vi "pathsConfig.vi"(0 "TDMS file out path IN":path=path "", 5 "Background out path IN":path=path "", 11 "Error IN":errorcluster caption="constante d'erreur") -> (15 "Error OUT":errorcluster caption="constante d'erreur")   [LabVIEW 2020]
panel:
  in  "OK":bool
  out "Background out path":path
  out "TDMS file out path":path
  # "PATHS CONFIGURATION"
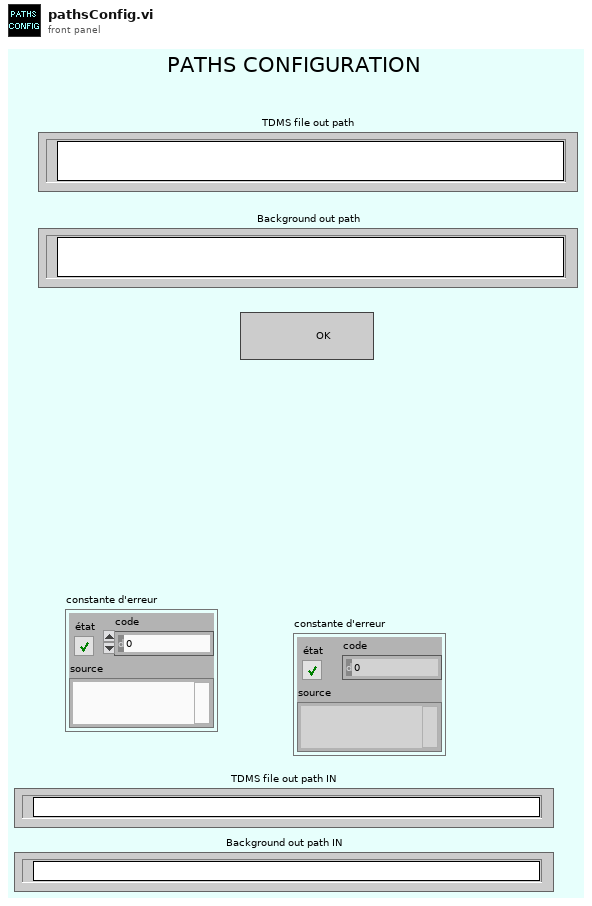
[diagram p1: front panel]
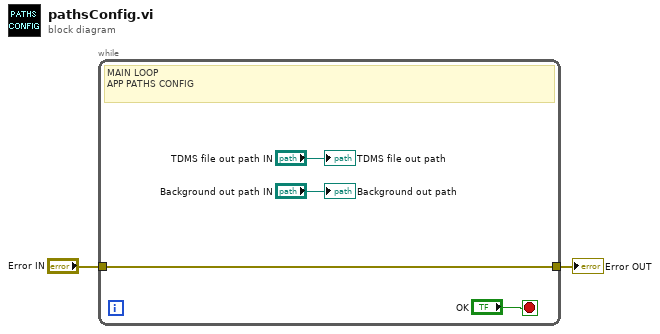
[diagram p0: block diagram]
diagram:
  n1 = while {
    tunnel: "Error IN" -> [w5]
    tunnel: [w5] -> w1
    stop <- "OK" stop-if-true
    # "MAIN LOOP\nAPP PATHS CONFIG"
    "Background out path" <- "Background out path IN"
    "TDMS file out path" <- "TDMS file out path IN"
  }
  "Error OUT" <- w1
